vi "SINGLE_v15_6.vi"() -> ()   [LabVIEW 2017]
uses:
  BERTTA/x64/Debug/BERTTA.dll
panel:
  in  "Log time interval (s)":dbl=15.0 caption="Time Target (s)"
  in  "Add comment":string
  in  "OK Button":bool
  out "Started:":string
  in  "SHUTDOWN":bool
  in  "MASTER CONTROL":bool
  in  "Tab Control":T1(tab)
  out "Output File":path caption="selected path"
  in  "Browse folder":path=path "C:/Users/shresplab/Desktop" caption="start path"
  in  "Read Seq":bool
  in  "Save Seq":bool
  in  "Configuration file":path caption="Filename"
  in  "OK Button 2":bool
  out "Boolean":bool
  in  "User (initials)":string
  in  "Project name":string
  in  "Description":string
  out "Led11 12":bool
  out "Target amount":dbl
  out "Scale weight":dbl
  out "Amount now":dbl
  out "Flow rate":dbl
  out "Time to target":dbl format="%<%H:%M:%S>t"
  out "Current step":dbl
  out "Target":dbl
  out "Amount now":dbl
  out "PUMP3":bool
  out "Led11 11":bool
  out "Amount now":dbl
  out "Target":dbl
  out "Current step":dbl
  out "Time to target":dbl format="%<%H:%M:%S>t"
  out "Flow rate":dbl
  out "Amount now":dbl
  out "Scale weight":dbl
  out "Target amount":dbl
  out "PUMP2":bool
  out "Target amount":dbl format="Target amount:        %#_g"
  out "Scale weight":dbl format="Scale weight:     %#_4g"
  out "Amount now":dbl format="Amount now:      %#_4g"
  out "Flow rate":dbl format="Flow rate:                   %#_4g"
  out "Time to target":dbl format="Time to target:     %<%H:%M:%S>t"
  out "Current step":dbl format="Current step:              %#_g"
  out "Target":dbl format="Target:                %#_4g"
  out "Amount now":dbl format="Amount now:    %#_4g"
  out "Led11 10":bool
  out "PUMP1":bool
  out "Sensor OK 6":bool
  out "Sensor OK 5":bool
  out "Sensor OK 4":bool
  out "Sensor OK 3":bool
  out "Tr":dbl format="Tr:              %#_4g"
  out "Tj in":dbl format="Tj in:        %#_4g"
  out "Tj out":dbl format="Tj out:        %#_4g"
  out "T set":dbl format="T set:          %#_4g"
  out "Current step":i32 format="Current step:  %.0f"
  out "RPM":dbl format="RPM:          %#_g"
  out "Torque 2":dbl format="Torque:      %#_g"
  out "T external 3":dbl format="T (S2):       %#_4g"
  out "Waveform Chart 5":dynamicdata(graph)
  out "Waveform Chart 6":dynamicdata(graph)
  out "Waveform Chart 7":dynamicdata(graph)
  in  "OK Button 11":bool=TRUE
  out "Table":string[][](table)=[["14.8.2017 18.06.59", "0,000000", "417,670000", "-0,150000", "1,000000", "22,220000", "23,366837", "23,574959", "23,985852", "23,690000", "240,000000", "4,000000", "0,000000", "397,000000", "-397,000000", "1,000000"], ["14.8.2017 18.07.06", "0,000000", "417,640000", "-0,120000", "1,000000", "22,220000", "23,763115", "23,906257", "23,985694", "23,680000", "240,000000", "4,000000", "0,000000", "397,000000", "-397,000000", "1,000000"], ["14.8.2017 18.07.13", "0,000000", "417,640000", "-0,120000", "1,000000", "22,220000", "23,965922", "24,013440", "23,984906", "23,670000", "240,000000", "4,100000", "3,000000", "397,000000", "-397,000000", "1,000000"], ["14.8.2017 18.07.21", "0,000000", "417,640000", "-0,120000", "1,000000", "22,220000", "23,943860", "23,900110", "23,987113", "23,670000", "240,000000", "4,000000", "0,000000", "397,000000", "-397,000000", "1,000000"], ["14.8.2017 18.07.28", "0,000000", "417,640000", "-0,120000", "1,000000", "22,220000", "23,736328", "23,600018", "23,989004", "23,660000", "240,000000", "4,000000", "0,000000", "397,000000", "-397,000000", "1,000000"], ["14.8.2017 18.07.36", "0,000000", "417,640000", "-0,120000", "1,000000", "22,220000", "23,480910", "23,324538", "23,991053", "23,660000", "240,000000", "4,000000", "0,000000", "397,000000", "-397,000000", "1,000000"], ["14.8.2017 18.07.43", "0,000000", "417,640000", "-0,120000", "2,000000", "22,220000", "23,195579", "23,008270", "23,999093", "23,650000", "240,000000", "4,000000", "0,000000", "397,000000", "-397,000000", "1,000000"], ["14.8.2017 18.07.51", "0,000000", "417,650000", "-417,650000", "1,000000", "22,220000", "22,862541", "22,649021", "24,003979", "23,650000", "240,000000", "4,000000", "0,000000", "397,000000", "-397,000000", "2,000000"], ["14.8.2017 18.07.58", "0,000000", "417,640000", "0,010000", "1,000000", "22,220000", "22,541353", "22,354878", "24,005398", "23,650000", "240,000000", "4,000000", "0,000000", "397,000000", "-397,000000", "1,000000"], ["14.8.2017 18.08.06", "0,000000", "417,640000", "0,010000", "1,000000", "22,220000", "22,347931", "22,253738", "24,007605", "23,640000", "240,000000", "4,100000", "0,000000", "397,000000", "-397,000000", "1,000000"], ["14.8.2017 18.08.13", "0,000000", "417,640000", "0,010000", "1,000000", "22,220000", "22,329030", "22,302102", "24,006028", "23,640000", "240,000000", "4,000000", "0,000000", "395,820000", "-395,820000", "1,000000"], ["14.8.2017 18.08.20", "0,000000", "417,640000", "0,010000", "1,000000", "22,220000", "22,466849", "22,511320", "24,002403", "23,630000", "240,000000", "4,000000", "0,000000", "395,830000", "-0,010000", "1,000000"], ["14.8.2017 18.08.28", "0,000000", "417,640000", "0,010000", "1,000000", "22,220000", "22,707062", "22,835101", "24,000984", "23,620000", "240,000000", "4,000000", "0,000000", "395,830000", "-0,010000", "1,000000"], ["14.8.2017 18.08.35", "0,000000", "417,640000", "0,010000", "1,000000", "22,220000", "23,054104", "23,232979", "24,001299", "23,600000", "240,000000", "4,000000", "0,000000", "395,830000", "-0,010000", "1,000000"], ["14.8.2017 18.08.43", "0,000000", "417,640000", "0,010000", "1,000000", "22,220000", "23,412371", "23,522793", "24,002560", "23,590000", "240,000000", "4,000000", "0,000000", "395,820000", "0,000000", "1,000000"], ["14.8.2017 18.08.51", "0,000000", "417,640000", "0,010000", "1,000000", "22,220000", "23,596247", "23,656125", "24,003821", "23,580000", "240,000000", "4,000000", "0,000000", "395,820000", "0,000000", "1,000000"]]
  out "LED_5":bool
  out "LED_4":bool
  in  "PAUSE/RUN 4":bool
  in  "TEMP RAMP":dbl[][](array[numeric])
  out "LED_3":bool
  out "LED_2":bool
  out "LED_1":bool
  out "LED_MANUAL":bool
  in  "Reset 6":bool
  in  "Manual/Ramp":bool=TRUE
  in  "Sensor selector":bool=TRUE
  in  "Tr/Tj mode selector":bool=TRUE
  out "LED STOP":bool
  in  "Failsafe":dbl=20.0 format="Failsafe temperature:            %#_g"
  out "Current temp":dbl format="Current temperature S1:       %#_4g"
  out "Sensor OK":bool
  out "T external 2":dbl format="Current temperature S2:       %#_4g"
  in  "OK Button 3":bool
  out "Waveform Chart":dynamicdata(graph)
  in  "X scales":i64(slide)=50 scale=0.0..100.0
  in  "PAUSE/RUN 9":bool=TRUE
  out "Led11 7":bool
  out "Led11 6":bool
  in  "PAUSE/RUN 3":bool
  in  "Tube select 3":u32(ring) items=["Big tube", "Double big tube", "Medium tube", "Small tube"]
  in  "Reset 8":bool
  out "Led11 9":bool
  in  "?":bool
  in  "Grams / min 3":dbl
  out "RPM 3":dbl format="%_4f"
  out "Flow rate (g/min) 3":dbl
  out "Scale reading 3":dbl
  out "Step amount now 3":dbl
  out "Total amount now 3":dbl
  out "Elapsed / step 3":dbl format="%<%H:%M:%S>t"
  out "Time to target 3":dbl format="%<%H:%M:%S>t"
  out "Led5 5":bool
  out "Led4 5":bool
  out "Led3 5":bool
  out "Led2 5":bool
  out "Led1 5":bool
  in  "PumpSeq 6":dbl[][](array[numeric])=[[0.0, 0.0, 0.0, 0.0, 0.0, 0.0, 0.0, 0.0, 0.0, 0.0], [0.0, 0.0, 0.0, 0.0, 0.0, 0.0, 0.0, 0.0, 0.0, 0.0], [0.0, 0.0, 0.0, 0.0, 0.0, 0.0, 0.0, 0.0, 0.0, 0.0], [0.0, 0.0, 0.0, 0.0, 0.0, 0.0, 0.0, 0.0, 0.0, 0.0], [0.0, 0.0, 0.0, 0.0, 0.0, 0.0, 0.0, 0.0, 0.0, 0.0], [0.0, 0.0, 0.0, 0.0, 0.0, 0.0, 0.0, 0.0, 0.0, 0.0], [0.0, 0.0, 0.0, 0.0, 0.0, 0.0, 0.0, 0.0, 0.0, 0.0], [0.0, 0.0, 0.0, 0.0, 0.0, 0.0, 0.0, 0.0, 0.0, 0.0], [0.0, 0.0, 0.0, 0.0, 0.0, 0.0, 0.0, 0.0, 0.0, 0.0], [0.0, 0.0, 0.0, 0.0, 0.0, 0.0, 0.0, 0.0, 0.0, 0.0]]
  out "Led11 8":bool
  in  "PAUSE/RUN 8":bool=TRUE
  out "Led11 7":bool
  out "Led11 6":bool
  in  "PAUSE/RUN 2":bool
  in  "Tube select 2":u32(ring) items=["Big tube", "Double big tube", "Medium tube", "Small tube"]
  out "Led11 7":bool
  in  "?":bool
  in  "Grams / min 2":dbl
  out "RPM 2":dbl format="%_4f"
  out "Flow rate (g/min) 2":dbl
  out "Scale reading 2":dbl
  out "Step amount now 2":dbl
  out "Total amount now 2":dbl
  out "Elapsed / step 2":dbl format="%<%H:%M:%S>t"
  out "Time to target 2":dbl format="%<%H:%M:%S>t"
  out "Led5 4":bool
  out "Led4 4":bool
  out "Led3 4":bool
  out "Led2 4":bool
  out "Led1 4":bool
  in  "PumpSeq 5":dbl[][](array[numeric])=[[0.0, 0.0, 0.0, 0.0, 0.0, 0.0, 0.0, 0.0, 0.0, 0.0], [0.0, 0.0, 0.0, 0.0, 0.0, 0.0, 0.0, 0.0, 0.0, 0.0], [0.0, 0.0, 0.0, 0.0, 0.0, 0.0, 0.0, 0.0, 0.0, 0.0], [0.0, 0.0, 0.0, 0.0, 0.0, 0.0, 0.0, 0.0, 0.0, 0.0], [0.0, 0.0, 0.0, 0.0, 0.0, 0.0, 0.0, 0.0, 0.0, 0.0], [0.0, 0.0, 0.0, 0.0, 0.0, 0.0, 0.0, 0.0, 0.0, 0.0], [0.0, 0.0, 0.0, 0.0, 0.0, 0.0, 0.0, 0.0, 0.0, 0.0], [0.0, 0.0, 0.0, 0.0, 0.0, 0.0, 0.0, 0.0, 0.0, 0.0], [0.0, 0.0, 0.0, 0.0, 0.0, 0.0, 0.0, 0.0, 0.0, 0.0], [0.0, 0.0, 0.0, 0.0, 0.0, 0.0, 0.0, 0.0, 0.0, 0.0]]
  out "Led11 6":bool
  in  "Reset 7":bool
  in  "PAUSE/RUN 7":bool=TRUE
  out "Led5 7":bool
  out "Led4 6":bool
  in  "PAUSE/RUN":bool
  in  "Tube select":u32(ring) items=["Big tube", "Double big tube", "Medium tube", "Small tube"]
  out "Led11 5":bool
  out "RPM":dbl format="RPM                      %_4f"
  out "Flow rate (g/min)":dbl format="Flow rate               %#_g"
  out "Scale reading":dbl format="Scale reading       %#_g"
  out "Step amount now":dbl format="Step amount       %#_g"
  out "Total amount now":dbl format="Total amount      %#_g"
  out "Elapsed / step":dbl format="Elapsed / step      %<%H:%M:%S>t"
  out "Time to target":dbl format="Time to target     %<%H:%M:%S>t"
  out "Led5 3":bool
  out "Led4 3":bool
  out "Led3 3":bool
  out "Led2 3":bool
  out "Led1 3":bool
  in  "PumpSeq 4":dbl[][](array[numeric])=[[0.0, 0.0, 0.0, 0.0, 0.0, 0.0, 0.0, 0.0, 0.0, 0.0], [0.0, 0.0, 0.0, 0.0, 0.0, 0.0, 0.0, 0.0, 0.0, 0.0], [0.0, 0.0, 0.0, 0.0, 0.0, 0.0, 0.0, 0.0, 0.0, 0.0], [0.0, 0.0, 0.0, 0.0, 0.0, 0.0, 0.0, 0.0, 0.0, 0.0], [0.0, 0.0, 0.0, 0.0, 0.0, 0.0, 0.0, 0.0, 0.0, 0.0], [0.0, 0.0, 0.0, 0.0, 0.0, 0.0, 0.0, 0.0, 0.0, 0.0], [0.0, 0.0, 0.0, 0.0, 0.0, 0.0, 0.0, 0.0, 0.0, 0.0], [0.0, 0.0, 0.0, 0.0, 0.0, 0.0, 0.0, 0.0, 0.0, 0.0], [0.0, 0.0, 0.0, 0.0, 0.0, 0.0, 0.0, 0.0, 0.0, 0.0], [0.0, 0.0, 0.0, 0.0, 0.0, 0.0, 0.0, 0.0, 0.0, 0.0]]
  in  "?":bool
  in  "Grams / min":dbl format="Manual g/min:  %#_g"
  out "Led11 4":bool
  in  "Reset 5":bool
  out "Waveform Chart 18":dynamicdata(graph)
  in  "OK Button 4":bool
  out "Waveform Chart 16":dynamicdata(graph)
  in  "OK Button 5":bool
  out "Waveform Chart 17":dynamicdata(graph)
  in  "OK Button 6":bool
  in  "PAUSE/RUN 5":bool
  in  "?":bool
  in  "Scale port":dbl=5.0
  out "Waveform Chart 15":dynamicdata(graph)
  in  "OK Button 8":bool
  out "RPM":dbl
  out "Torque":dbl
  out "Waveform Chart 4":dynamicdata(graph)
  in  "OK Button 7":bool
  in  "CDAQ 1 Temp Control":tag="cDAQ9188XT-1C3BF12Mod1"
  in  "CDAQ PAM Control":tag="cDAQ9188XT-1C3BF12Mod7"
  in  "PORT PUMP2":i32 format="PUMP 2 PORT:  %.0f"
  in  "PORT PUMP3":i32 format="PUMP 3 PORT:  %.0f"
  in  "PORT PUMP1":i32 format="PUMP 1 PORT:  %.0f"
  in  "Save PortDev":bool
  in  "LAUDA":i32 format="LAUDA 1 PORT:  %.0f"
  in  "HEIDOLPH":i32 format="HEIDOLPH 1 PORT:  %.0f"
  in  "SCALE1":i32 format="SCALE 1 PORT:  %.0f"
  in  "SCALE2":i32 format="SCALE 2 PORT:  %.0f"
  in  "SCALE 3":i32 format="SCALE 3 PORT:  %.0f"
  # "Sensor:"
  # "Control:"
  # "PUMP & SCALE 3"
  # "STEP"
  # "TOTAL"
  # "PUMP & SCALE 2"
  # "STEP"
  # "TOTAL"
  # "PUMP & SCALE 1"
  # "STEP"
  # "TOTAL"
  # "MANUAL"
  # "RAMP"
  # "Temp Target       Time Target          Wait Time"
  # "STOP"
  # "g              min"
  # "g              min"
  # "g              min"
  # "PAM control"
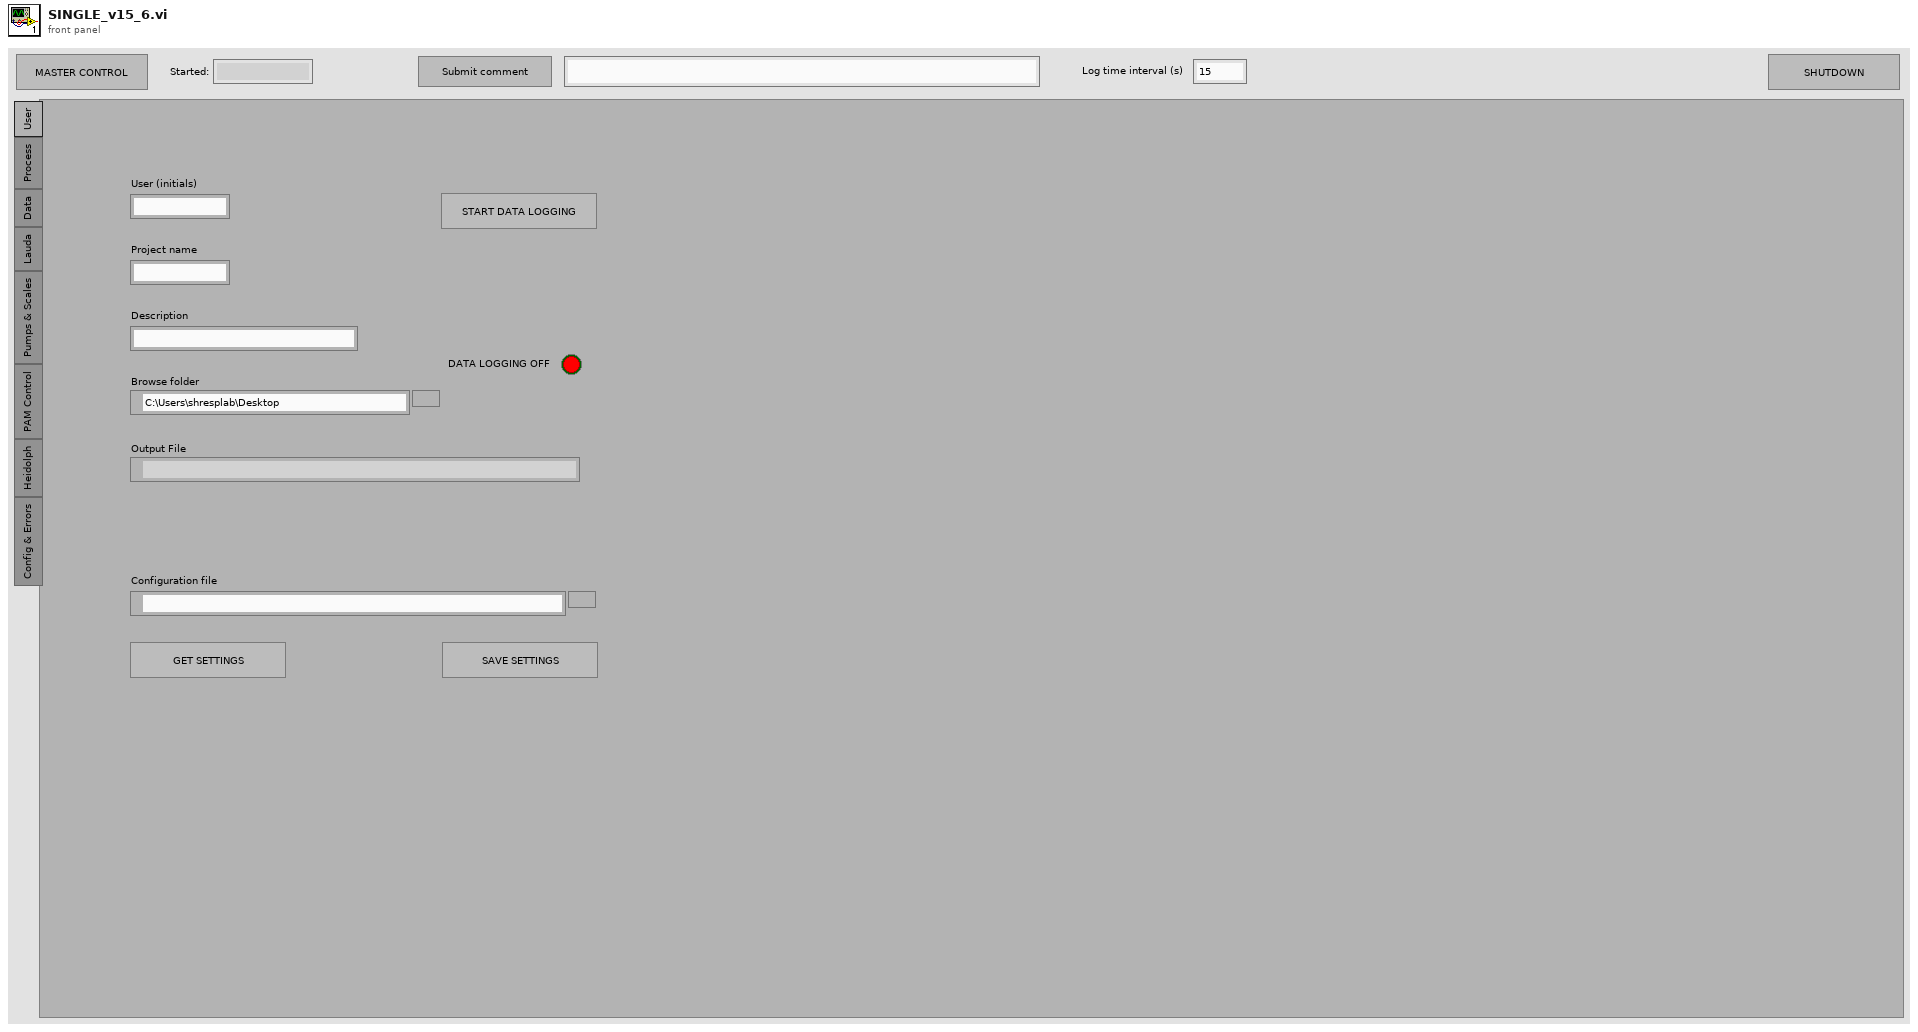
[diagram p1: front panel]
types:
  T1 = enum32{"User", "Process", "Data", "Lauda", "Pumps & Scales", "PAM Control", "Heidolph", "Config & Errors"}
diagram:
  n1 = while {
    i -> [w192]
    stop <- FALSE stop-if-true
    w131 = i64 1000 ("y")
    # "SCALE & PUMP 3"
    n2 = Not(x="MASTER CONTROL") -> (.not. x?=w227:bool)
    n3 = Boolean To (0,1)(Boolean="PAUSE/RUN 7") -> (0, 1=w27:i16)
    n4 = Boolean To (0,1)(Boolean="PAUSE/RUN 8") -> (0, 1=w26:i16)
    n5 = Boolean To (0,1)(Boolean="PAUSE/RUN 9") -> (0, 1=w25:i16)
    n6 = control-ref of="This VI"() -> (w123:refnum<vi>)
    n7 = Multiply(x="X scales", y=w131) -> (x*y=w132:i64)
    n8 = Boolean To (0,1)(Boolean=w227) -> (0, 1=w228:i16)
    n9 = call "RampCTRL_1.vi"("TEMP RAMP"="TEMP RAMP", "Reset 6"="Reset 6") -> ("Array"=w153:dbl[], "Array 2"=w154:dbl[], "Array 3"=w155:dbl[])  [unwired: 7 in]
    n10 = Add(x=w132, y=w131) -> (x+y=w43:i64)
    n11 = for {
      N: w228 -> [_]
      n12 = Get Date/Time String(want seconds? (F)=TRUE) -> (time string=→"Started:":string)  [unwired: 2 in, 1 out]
    }
    n13 = Boolean To (0,1)(Boolean="Sensor selector") -> (0, 1=w148:i16)
    n14 = feedback #1() -> (w130:i64)  [unwired: 1 in]
    n15 = feedback-in #1(w43) -> ()
    n16 = call "shutdown sequence.vi"("SHUTDOWN"="SHUTDOWN", "VI in"=w123) -> ()  [unwired: 10 in]
    n17 = Boolean To (0,1)(Boolean="SHUTDOWN") -> (0, 1=w122:i16)
    n18 = Boolean To (0,1)(Boolean="Reset 6") -> (0, 1=w165:i16)
    n19 = Not Equal?(x=w130, y=w43) -> (x != y?=w129:bool)
    n20 = property on="Waveform Chart" class="WFChart (strict)"() -> ("History Data"=w134:dynamicdata[])  [unwired: 2 in, 2 out]
    n21 = Boolean To (0,1)(Boolean=w129) -> (0, 1=w127:i16)
    n22 = Array Size(array=w134) -> (size(s)=w128:i32)
    n23 = call "ReadMoxa8.vi"("PORT 1"="LAUDA", "PORT 2"="HEIDOLPH", "PORT 3"="SCALE1", "PORT 4"="SCALE2", "PORT 5"="SCALE 3", "PORT 6"="PORT PUMP1", "PORT 7"="PORT PUMP2", "PORT 8"="PORT PUMP3", "enable1"=w27, "enable2"=w26, "enable3"=w25) -> ("params"=w29:dbl[])  [unwired: 8 in]
    n24 = Boolean To (0,1)(Boolean="Tr/Tj mode selector") -> (0, 1=w149:i16)
    n25 = call "SensorMode1.vi"("Numeric"=w148, "Numeric 2"=w149) -> ("Sensor OK 4"=→"Sensor OK 4":bool, "Sensor OK 5"=→"Sensor OK 5":bool, "Sensor OK 6"=→"Sensor OK 6":bool, "Sensor OK 3"=→"Sensor OK 3":bool)  [unwired: 6 in]
    n26 = for {
      N: w127 -> [_]
      tunnel: w128 -> [w247]
      tunnel: w43 -> [w246]
      n27 = Add(x=w247, y=w246) -> (x+y=w245:i64)
      n28 = property on="Waveform Chart" class="WFChart (strict)"("XScale.Maximum"=w245) -> ()  [unwired: 2 in, 2 out]
    }
    n29 = Boolean To (0,1)(Boolean="Manual/Ramp") -> (0, 1=w163:i16)
    n30 = And(x="MASTER CONTROL", y="PAUSE/RUN 4") -> (x .and. y?=w162:bool)
    n31 = Build Array("LAUDA", "HEIDOLPH", "SCALE1", "SCALE2", "SCALE 3", "PORT PUMP1", "PORT PUMP2", "PORT PUMP3") -> (w138:i32[])
    n32 = Boolean To (0,1)(Boolean=w162) -> (0, 1=w161:i16)
    n33 = call "LaudaDAQ.vi"("device name"="CDAQ 1 Temp Control") -> (1:"Tj out"=→"Tj out":dbl, "data"=w221:dynamicdata, "Sensor OK"=→"Sensor OK":bool, 4:"Tj out"=→"Tj in":dbl, "T external 2"=w124:dbl)  [unwired: 5 in, 1 out]
    "T external 2" <- w124
    "T external 3" <- w124
    n34 = Boolean To (0,1)(Boolean="Save PortDev") -> (0, 1=w195:i16)
    n35 = for {
      N: w195 -> [_]
      tunnel: w138 -> [w293]
      tunnel: "Save PortDev" -> [w294]
      n36 = call "Convert to Dynamic Data"("Array"=w293) -> ("Dynamic Data Type"=w292:dynamicdata)  [unwired: 3 in]
      n37 = call "Write To Measurement File3"("Signals"=w292, "Reset"=w294) -> ()  [unwired: 15 in, 3 out]
    }
    n38 = Less?(x=w192, y=1.0) -> (x < y?=w190:bool)
    n39 = call "HEI_Data_single.vi"("params"=w29) -> ("RPM"=w12:dbl, "Dynamic Data"=w16:dynamicdata, "Torque"=→"Torque" →"Torque 2":dbl)  [unwired: 16 in]
    "Waveform Chart 4" <- w16
    "RPM" <- w12
    "Waveform Chart 6" <- w16
    "RPM" <- w12
    n40 = Boolean To (0,1)(Boolean=w190) -> (0, 1=w191:i16)
    n41 = Equal?(x=w12, y=0.0) -> (x = y?=w14:bool)
    n42 = Boolean To (0,1)(Boolean=w14) -> (0, 1=w13:i16)
    n43 = call "Fail_Clock_1.vi"("fail"=w13) -> ("Trigger"=w11:dbl)  [unwired: 10 in]
    n44 = call "Ramp_Lauda_v3.vi"("manual"=w163, "Tr_Tj"=w149, "shutdown"=w122, "S1_S2"=w148, "Tr"=w29, "T_fail"="Failsafe", "fail"=w11, "enable"=w161, "time_set"=w154, "reset"=w165, "time_wait"=w153, "T_S2"=w124, "port"="LAUDA", "T_sp"=w155) -> ("LED_1"=→"LED_1":bool, "LED_manual"=→"LED_MANUAL":bool, "LED_2"=→"LED_2":bool, "step"=w141:dbl, "LED_stop"=→"LED STOP":bool, "LED_3"=→"LED_3":bool, "LED 4"=→"LED_4":bool, "LED 5"=→"LED_5":bool, "setpoint"=w30:dbl, "Tr_out"=w160:dbl, "T int"=w159:dbl)  [unwired: 1 in, 2 out]
    "Tr" <- w160
    "T set" <- w30
    "Current temp" <- w160
    n45 = Add(x=w141, y=1.0) -> (x+y=→"Current step":dbl)
    n46 = Merge Signals(w30, w160, w159, w221) -> (w37:dynamicdata)
    "Waveform Chart" <- w37
    "Waveform Chart 5" <- w37
    n47 = for {
      N: w191 -> [_]
      tunnel: w190 -> [w287]
      n48 = while {
        tunnel: [w290] -> w286
        tunnel: w287 -> [w288]
        stop <- w291 stop-if-true
        n49 = call "Read From Measurement File2"("Enable"=TRUE, "Reset"=w288) -> ("Signals"=w290:dynamicdata, "EOF?"=w291:bool)  [unwired: 4 in, 4 out]
      }
      n50 = call "Convert from Dynamic Data2"("Dynamic Data Type"=w286) -> ("Array"=w269:dbl[])  [unwired: 3 in]
      n51 = Index Array(array=w269, index=0) -> (element=w279:dbl)
      n52 = Index Array(array=w269, index=1) -> (element=w278:dbl)
      n53 = Index Array(array=w269, index=2) -> (element=w277:dbl)
      n54 = Index Array(array=w269, index=3) -> (element=w276:dbl)
      n55 = Index Array(array=w269, index=4) -> (element=w275:dbl)
      n56 = Index Array(array=w269, index=5) -> (element=w270:dbl)
      n57 = Index Array(array=w269, index=6) -> (element=w272:dbl)
      n58 = Index Array(array=w269, index=7) -> (element=w271:dbl)
      n59 = property on="LAUDA" class="DigNum (strict)"("Val(Sgnl)"=w279) -> ()  [unwired: 2 in, 2 out]
      n60 = property on="HEIDOLPH" class="DigNum (strict)"("Val(Sgnl)"=w278) -> ()  [unwired: 2 in, 2 out]
      n61 = property on="SCALE1" class="DigNum (strict)"("Val(Sgnl)"=w277) -> ()  [unwired: 2 in, 2 out]
      n62 = property on="SCALE2" class="DigNum (strict)"("Val(Sgnl)"=w276) -> ()  [unwired: 2 in, 2 out]
      n63 = property on="SCALE 3" class="DigNum (strict)"("Val(Sgnl)"=w275) -> ()  [unwired: 2 in, 2 out]
      n64 = property on="PORT PUMP1" class="DigNum (strict)"("Val(Sgnl)"=w270) -> ()  [unwired: 2 in, 2 out]
      n65 = property on="PORT PUMP2" class="DigNum (strict)"("Val(Sgnl)"=w272) -> ()  [unwired: 2 in, 2 out]
      n66 = property on="PORT PUMP3" class="DigNum (strict)"("Val(Sgnl)"=w271) -> ()  [unwired: 2 in, 2 out]
    }
    n67 = Boolean To (0,1)(Boolean="OK Button 3") -> (0, 1=w202:i16)
    n68 = for {
      N: w202 -> [_]
      n69 = property on="Waveform Chart" class="WFChart (strict)"("History Data"=dynamicdata[] []) -> ()  [unwired: 2 in, 2 out]
    }
    n70 = Boolean To (0,1)(Boolean="OK Button 4") -> (0, 1=w200:i16)
    n71 = for {
      N: w200 -> [_]
      n72 = property on="Waveform Chart 18" class="WFChart (strict)"("History Data"=dynamicdata[] []) -> ()  [unwired: 2 in, 2 out]
    }
    n73 = Boolean To (0,1)(Boolean="OK Button 5") -> (0, 1=w147:i16)
    n74 = for {
      N: w147 -> [_]
      n75 = property on="Waveform Chart 16" class="WFChart (strict)"("History Data"=dynamicdata[] []) -> ()  [unwired: 2 in, 2 out]
    }
    n76 = call "IsmaCTRL_single.vi"("FR_manual"="Grams / min", "tube selector"="Tube select", "Manual"="?", "Reset"="Reset 5", "Pause"="PAUSE/RUN", "Setpoint_W   /   Setpoint_T"="PumpSeq 4", "Enable"="MASTER CONTROL", "Scale"=w29) -> ("Boolean 9"=→"Led11 5" →"Led11 10":bool, "Boolean"=→"Led1 3":bool, "Boolean 2"=→"Led2 3":bool, "Total target"=→"Target":dbl, "Boolean 3"=→"Led3 3":bool, "Boolean 4"=→"Led4 3":bool, "lastAmount"=→"Step amount now":dbl, "step"=→"Current step":dbl, "Boolean 5"=→"Led5 3":bool, "Boolean 6"=→"Led4 6":bool, "Boolean 7"=→"Led5 7":bool, "FR"=w105:dbl, "RPM"=w33:dbl, "Weight"=w101:dbl, "elapsed"=→"Elapsed / step":dbl, "time_to_target"=→"Time to target" →"Time to target":dbl, "pumpCTRL"=w117:dbl, "Target_step"=→"Target amount":dbl, "Boolean 8"=w109:bool)  [unwired: 1 out]
    "Flow rate" <- w105
    "Scale weight" <- w101
    "Led11 4" <- w109
    "Scale reading" <- w101
    "Flow rate (g/min)" <- w105
    "RPM" <- w33
    n77 = Boolean To (0,1)(Boolean="OK Button 6") -> (0, 1=w145:i16)
    n78 = for {
      N: w145 -> [_]
      n79 = property on="Waveform Chart 17" class="WFChart (strict)"("History Data"=dynamicdata[] []) -> ()  [unwired: 2 in, 2 out]
    }
    n80 = Multiply(x=w101, y=-1.0 ("x")) -> (x*y=→"Amount now" →"Amount now" →"Total amount now":dbl)
    n81 = And(x="PAUSE/RUN", y=w109) -> (x .and. y?=w180:bool)
    n82 = feedback #2() -> (w181:bool)  [unwired: 1 in]
    n83 = feedback-in #2(w180) -> ()
    n84 = Greater?(x=w117, y=70.0) -> (0:→"PUMP1":bool)
    n85 = Not Equal?(x=w181, y=w180) -> (x != y?=w179:bool)
    n86 = Boolean To (0,1)(Boolean=w179) -> (0, 1=w178:i16)
    n87 = for {
      N: w178 -> [_]
      n88 = property on="PAUSE/RUN" class="Bool (strict)"("Val(Sgnl)"=FALSE ("Value (Signaling)")) -> ()  [unwired: 2 in, 2 out]
    }
    n89 = Merge Signals(w101, w105) -> (w3:dynamicdata)
    "Waveform Chart 17" <- w3
    n90 = Boolean To (0,1)(Boolean="OK Button 7") -> (0, 1=w198:i16)
    n91 = for {
      N: w198 -> [_]
      n92 = property on="Waveform Chart 4" class="WFChart (strict)"("History Data"=dynamicdata[] []) -> ()  [unwired: 2 in, 2 out]
    }
    n93 = call "IsmaCTRL_2_single.vi"("FR_manual"="Grams / min 2", "tube selector"="Tube select 2", "Manual"="?", "Reset"="Reset 7", "Pause"="PAUSE/RUN 2", "Setpoint_W   /   Setpoint_T"="PumpSeq 5", "Enable"="MASTER CONTROL", "Scale"=w29) -> ("Boolean 9"=→"Led11 7" →"Led11 11":bool, "Boolean"=→"Led1 4":bool, "Boolean 2"=→"Led2 4":bool, "Total target"=→"Target":dbl, "Boolean 3"=→"Led3 4":bool, "Boolean 4"=→"Led4 4":bool, "lastAmount"=→"Amount now" →"Step amount now 2":dbl, "step"=→"Current step":dbl, "Boolean 5"=→"Led5 4":bool, "Boolean 6"=→"Led11 6":bool, "Boolean 7"=→"Led11 7":bool, "FR"=w88:dbl, "RPM"=w32:dbl, "Weight"=w89:dbl, "elapsed"=→"Elapsed / step 2":dbl, "time_to_target"=→"Time to target" →"Time to target 2":dbl, "pumpCTRL"=w82:dbl, "Target_step"=→"Target amount":dbl, "Boolean 8"=w72:bool)  [unwired: 1 out]
    "Scale weight" <- w89
    "Flow rate" <- w88
    "Led11 6" <- w72
    "Scale reading 2" <- w89
    "Flow rate (g/min) 2" <- w88
    "RPM 2" <- w32
    n94 = Boolean To (0,1)(Boolean="OK Button 8") -> (0, 1=w187:i16)
    n95 = for {
      N: w187 -> [_]
      n96 = property on="Waveform Chart 15" class="WFChart (strict)"("History Data"=dynamicdata[] []) -> ()  [unwired: 2 in, 2 out]
    }
    n97 = Merge Signals(w89, w88) -> (w2:dynamicdata)
    "Waveform Chart 18" <- w2
    n98 = Multiply(x=w89, y=-1.0) -> (x*y=→"Amount now" →"Total amount now 2":dbl)
    n99 = And(x="PAUSE/RUN 2", y=w72) -> (x .and. y?=w174:bool)
    n100 = Greater?(x=w82, y=70.0) -> (0:→"PUMP2":bool)
    n101 = feedback #3() -> (w175:bool)  [unwired: 1 in]
    n102 = feedback-in #3(w174) -> ()
    n103 = Not Equal?(x=w175, y=w174) -> (x != y?=w173:bool)
    n104 = Boolean To (0,1)(Boolean=w173) -> (0, 1=w172:i16)
    n105 = for {
      N: w172 -> [_]
      n106 = property on="PAUSE/RUN 2" class="Bool (strict)"("Val(Sgnl)"=FALSE ("Value (Signaling)")) -> ()  [unwired: 2 in, 2 out]
    }
    n107 = call "IsmaCTRL_3_single.vi"("FR_manual"="Grams / min 3", "tube selector"="Tube select 3", "Manual"="?", "Reset"="Reset 8", "Pause"="PAUSE/RUN 3", "Setpoint_W   /   Setpoint_T"="PumpSeq 6", "Enable"="MASTER CONTROL", "Scale"=w29) -> ("Boolean 9"=→"Led11 9" →"Led11 12":bool, "Boolean"=→"Led1 5":bool, "Boolean 2"=→"Led2 5":bool, "Total target"=→"Target":dbl, "Boolean 3"=→"Led3 5":bool, "Boolean 4"=→"Led4 5":bool, "lastAmount"=→"Amount now" →"Step amount now 3":dbl, "step"=→"Current step":dbl, "Boolean 5"=→"Led5 5":bool, "Boolean 6"=→"Led11 6":bool, "Boolean 7"=→"Led11 7":bool, "FR"=w58:dbl, "RPM"=w31:dbl, "Weight"=w57:dbl, "elapsed"=→"Elapsed / step 3":dbl, "time_to_target"=→"Time to target" →"Time to target 3":dbl, "pumpCTRL"=w63:dbl, "Target_step"=→"Target amount":dbl, "Boolean 8"=w48:bool)  [unwired: 1 out]
    "Scale weight" <- w57
    "Flow rate" <- w58
    "Led11 8" <- w48
    "Scale reading 3" <- w57
    "Flow rate (g/min) 3" <- w58
    "RPM 3" <- w31
    n108 = call "WriteMoxa8.vi"("PORT LAUDA 1"="LAUDA", "DATA LAUDA 1"=w30, "enable2"=w26, "DATA ISMA 1"=w33, "DATA ISMA 2"=w32, "enable1"=w27, "PORT ISMA 1"="PORT PUMP1", "DATA ISMA 3"=w31, "PORT ISMA 2"="PORT PUMP2", "PORT ISMA 3"="PORT PUMP3", "enable3"=w25) -> ()  [unwired: 5 in]
    n109 = Multiply(x=w57, y=-1.0) -> (x*y=→"Amount now" →"Total amount now 3":dbl)
    n110 = Merge Signals(w101, w89, w57) -> (→"Waveform Chart 7":dynamicdata)
    n111 = Greater?(x=w63, y=70.0) -> (0:→"PUMP3":bool)
    n112 = And(x="MASTER CONTROL", y=w48) -> (x .and. y?=w168:bool)
    n113 = Merge Signals(w57, w58) -> (w1:dynamicdata)
    "Waveform Chart 16" <- w1
    n114 = feedback #4() -> (w169:bool)  [unwired: 1 in]
    n115 = feedback-in #4(w168) -> ()
    n116 = Not Equal?(x=w169, y=w168) -> (x != y?=w167:bool)
    n117 = Boolean To (0,1)(Boolean=w167) -> (0, 1=w166:i16)
    n118 = for {
      N: w166 -> [_]
      n119 = property on="PAUSE/RUN 3" class="Bool (strict)"("Val(Sgnl)"=FALSE ("Value (Signaling)")) -> ()  [unwired: 2 in, 2 out]
    }
    n120 = call "Convert to Dynamic Data6"() -> ("Dynamic Data Type"=w36:dynamicdata)  [unwired: 4 in]
    n121 = call "Convert to Dynamic Data4"("2D Array"="PumpSeq 6") -> ("Dynamic Data Type"=w208:dynamicdata)  [unwired: 3 in]
    n122 = call "Convert to Dynamic Data3"("2D Array"="PumpSeq 5") -> ("Dynamic Data Type"=w209:dynamicdata)  [unwired: 3 in]
    n123 = call "Convert to Dynamic Data2"("2D Array"="PumpSeq 4") -> ("Dynamic Data Type"=w211:dynamicdata)  [unwired: 3 in]
    n124 = Merge Signals(w36, w208, w209, w211) -> (w210:dynamicdata)
    n125 = Boolean To (0,1)(Boolean="Save Seq") -> (0, 1=w207:i16)
    n126 = for {
      N: w207 -> [_]
      tunnel: w210 -> [w326]
      tunnel: "Configuration file" -> [w327]
      tunnel: "Save Seq" -> [w325]
      n127 = call "Write To Measurement File2"("Signals"=w326, "Reset"=w325, "Filename"=w327) -> ()  [unwired: 14 in, 3 out]
    }
    n128 = Boolean To (0,1)(Boolean="Read Seq") -> (0, 1=w206:i16)
    n129 = for {
      N: w206 -> [_]
      tunnel: "Configuration file" -> [w312]
      tunnel: "Read Seq" -> [w311]
      n130 = while {
        tunnel: [w324] -> w320
        tunnel: w312 -> [w323]
        tunnel: w311 -> [w321]
        stop <- w322 stop-if-true
        n131 = call "Read From Measurement File"("Filename"=w323, "Reset"=w321) -> ("Signals"=w324:dynamicdata, "EOF?"=w322:bool)  [unwired: 4 in, 4 out]
      }
      n132 = call "Convert from Dynamic Data"("Dynamic Data Type"=w320) -> ("Array"=w315:dbl[][])  [unwired: 3 in]
      n133 = Array Subset(array=w315, index (row)=20 ("index"), length (row)=10 ("length")) -> (w308:dbl[][])  [unwired: 2 in]
      n134 = Array Subset(array=w315, index (row)=10 ("index"), length (row)=10 ("length")) -> (w309:dbl[][])  [unwired: 2 in]
      n135 = Array Subset(array=w315, index (row)=30 ("index"), length (row)=8 ("length")) -> (w310:dbl[][])  [unwired: 2 in]
      n136 = property on="PumpSeq 6" class="Arr (strict)"("Val(Sgnl)"=w309) -> ()  [unwired: 2 in, 2 out]
      n137 = property on="PumpSeq 4" class="Arr (strict)"("Val(Sgnl)"=w310) -> ()  [unwired: 2 in, 2 out]
      n138 = property on="PumpSeq 5" class="Arr (strict)"("Val(Sgnl)"=w308) -> ()  [unwired: 2 in, 2 out]
    }
    n139 = Merge Signals(w3, w2, w1) -> (w222:dynamicdata)
    n140 = Merge Signals(w37, w222, w16) -> (w189:dynamicdata)
    n141 = Boolean To (0,1)(Boolean="PAUSE/RUN 5") -> (0, 1=w151:i16)
    n142 = for {
      N: w151 -> [_]
      tunnel: "MASTER CONTROL" -> [w251]
      tunnel: "PAUSE/RUN 5" -> [w250]
      n143 = And(x=w250, y="?") -> (x .and. y?=w259:bool)
      n144 = dll-call lib="C:/Users/shresplab/OneDrive - Kemira Oyj/Documents/GitHub/Bertta/BERTTA/x64/Debug/BERTTA.dll" fn="mettler"("port"="Scale port", "msg"=1) -> ("return type"=w253:dbl)  [unwired: 5 in, 2 out]
      n145 = And(x=w251, y=w259) -> (x .and. y?=w256:bool)
      n146 = Initialize Array(FALSE, 1 ("dimension size")) -> (w258:bool[])
      n147 = Replace Array Subset(array=w258, new element=w256, index=0) -> (w255:bool[])
      n148 = call "Convert to Dynamic Data5"("Double"=w253) -> ("Dynamic Data Type"=→"Waveform Chart 15":dynamicdata)  [unwired: 3 in]
      n149 = call "DAQ Assistant"("data"=w255, "device name"="CDAQ PAM Control") -> ()  [unwired: 16 in, 2 out]
    }
    n150 = call "filenameparser_09.vi"("Description"="Description", "start path"="Browse folder", "Project name"="Project name", "User (initials)"="User (initials)", "OK Button in"="OK Button 2") -> ("appended path 2"=w196:path, "appended path"=w224:path)  [unwired: 4 in, 1 out]
    "Output File" <- w196
    n151 = feedback #5() -> (w5:i32)  [unwired: 1 in]
    n152 = Boolean To (0,1)(Boolean="OK Button") -> (0, 1=w223:i16)
    n153 = Equal?(x=1.0, y=w5) -> (x = y?=w8:bool)
    n154 = call "Elapsed Time"("Time Target (s)"="Log time interval (s)", "Reset"=w8) -> ("Time has Elapsed"=w9:bool)  [unwired: 10 in, 7 out]
    n155 = for {
      N: w223 -> [_]
      tunnel: w224 -> [w300]
      w304 = " " ("string")
      n156 = property on="Add comment" class="Str"("Val(Sgnl)"="" ("Value (Signaling)")) -> ()  [unwired: 2 in, 2 out]
      n157 = Get Date/Time String(want seconds? (F)=TRUE) -> (date string=w307:string, time string=w305:string)  [unwired: 2 in]
      n158 = Concatenate Strings(w307, w304, w305, w304, "Add comment") -> (w303:string)
      n159 = feedback #6() -> (w302:string[])  [unwired: 1 in]
      n160 = Build Array (concatenate)(w302, w303) -> (w301:string[])
      n161 = feedback-in #6(w301) -> ()
      n162 = Write to Text File(file (use dialog)=w300, text=w301) -> ()  [unwired: 2 in, 3 out]
    }
    n163 = Boolean To (0,1)(Boolean=w9) -> (0, 1=w10:i16)
    n164 = Boolean To (0,1)(Boolean="OK Button 11") -> (0, 1=w34:i16)
    n165 = for {
      N: w10 -> [_]
      tunnel: "OK Button 2" -> [w238]
      tunnel: w196 -> [w237]
      tunnel: w189 -> [w236]
      tunnel: w34 -> [w235]
      tunnel: [w233] -> w6
      i -> [w233]
      n166 = call "Header Names Single.vi"("Dynamic Data"=w236) -> ("Signals Out"=w234:dynamicdata)  [unwired: 10 in]
      n167 = call "Write To Measurement File"("Signals"=w234, "Enable"=w238, "Filename"=w237) -> ()  [unwired: 14 in, 3 out]
      n168 = for {
        N: w235 -> [_]
        tunnel: w236 -> [w239]
        n169 = call "Build Table"("Include time data"=TRUE, "Signals"=w239) -> ("Table"=w243:string[][])  [unwired: 3 in, 6 out]
        n170 = Delete From Array(array=w243, length=13, index (col)=0 ("index (row)")) -> (array with subset deleted=→"Table":string[][])  [unwired: 1 in, 1 out]
      }
    }
    n171 = feedback-in #5(w6) -> ()
    "Boolean" <- "OK Button 2"
  }
